vi "test Update Discrete Bit Field by Data Type.vi"(8 "error in (no error)":errorcluster, 11 "TestCase in":refnum<class "Discrete.lvclass">) -> (0 "error out":errorcluster, 3 "TestCase out":refnum<class "Discrete.lvclass">)   [LabVIEW 2027, in "Discrete.lvclass"]
uses:
  Discrete.lvclass
  6e1d2ac8-71cc-41db-b083-493d6063b283.vi
  b2aaa37d-0322-432e-9b3a-1a1fc6048de9.vi
  93c23f9b-5cd3-4544-9818-cc1d3354fe3b.vi
  d5bea4d0-148e-442b-ba51-e57cfb69b26e.vi
  0a8c8d56-0a15-4b3b-b00b-207fe3918b86.vi
  2c49008a-66d3-44d5-b62f-9e3dae6c920e.vi
  4d7c551b-64cf-497b-b044-69caef92442e.vi
  8e8a66e8-53e0-4356-8f39-caffdde6a543.vi
  751b3aa0-6cbc-42a9-8f45-cac4046d3a07.vi
  c0b90d40-c6d8-43ae-bb04-9b0646120204.vi
  7f187975-33e1-49fe-bcee-bbe8f41f89f8.vi
  20f2966f-f599-41d1-9ff8-715ba5da5165.vi
  6e1d2ac8-71cc-41db-b083-493d6063b283.vi/9935dc85-f143-411c-b80b-16b6c96eb14a.vi
  6e1d2ac8-71cc-41db-b083-493d6063b283.vi/b24d9be9-5807-4d59-88b8-dc532f996cb3.vi
  6e1d2ac8-71cc-41db-b083-493d6063b283.vi/e4a2156f-f189-4bbd-8a3a-9da1a7e591f8.vi
  b2aaa37d-0322-432e-9b3a-1a1fc6048de9.vi/9935dc85-f143-411c-b80b-16b6c96eb14a.vi
  b2aaa37d-0322-432e-9b3a-1a1fc6048de9.vi/b24d9be9-5807-4d59-88b8-dc532f996cb3.vi
  b2aaa37d-0322-432e-9b3a-1a1fc6048de9.vi/e4a2156f-f189-4bbd-8a3a-9da1a7e591f8.vi
  93c23f9b-5cd3-4544-9818-cc1d3354fe3b.vi/9935dc85-f143-411c-b80b-16b6c96eb14a.vi
  93c23f9b-5cd3-4544-9818-cc1d3354fe3b.vi/b24d9be9-5807-4d59-88b8-dc532f996cb3.vi
  93c23f9b-5cd3-4544-9818-cc1d3354fe3b.vi/e4a2156f-f189-4bbd-8a3a-9da1a7e591f8.vi
  d5bea4d0-148e-442b-ba51-e57cfb69b26e.vi/9935dc85-f143-411c-b80b-16b6c96eb14a.vi
  d5bea4d0-148e-442b-ba51-e57cfb69b26e.vi/b24d9be9-5807-4d59-88b8-dc532f996cb3.vi
  d5bea4d0-148e-442b-ba51-e57cfb69b26e.vi/e4a2156f-f189-4bbd-8a3a-9da1a7e591f8.vi
  0a8c8d56-0a15-4b3b-b00b-207fe3918b86.vi/9935dc85-f143-411c-b80b-16b6c96eb14a.vi
  0a8c8d56-0a15-4b3b-b00b-207fe3918b86.vi/b24d9be9-5807-4d59-88b8-dc532f996cb3.vi
  0a8c8d56-0a15-4b3b-b00b-207fe3918b86.vi/e4a2156f-f189-4bbd-8a3a-9da1a7e591f8.vi
  2c49008a-66d3-44d5-b62f-9e3dae6c920e.vi/9935dc85-f143-411c-b80b-16b6c96eb14a.vi
  2c49008a-66d3-44d5-b62f-9e3dae6c920e.vi/b24d9be9-5807-4d59-88b8-dc532f996cb3.vi
  2c49008a-66d3-44d5-b62f-9e3dae6c920e.vi/e4a2156f-f189-4bbd-8a3a-9da1a7e591f8.vi
  4d7c551b-64cf-497b-b044-69caef92442e.vi/9935dc85-f143-411c-b80b-16b6c96eb14a.vi
  4d7c551b-64cf-497b-b044-69caef92442e.vi/b24d9be9-5807-4d59-88b8-dc532f996cb3.vi
  4d7c551b-64cf-497b-b044-69caef92442e.vi/e4a2156f-f189-4bbd-8a3a-9da1a7e591f8.vi
  8e8a66e8-53e0-4356-8f39-caffdde6a543.vi/9935dc85-f143-411c-b80b-16b6c96eb14a.vi
  8e8a66e8-53e0-4356-8f39-caffdde6a543.vi/b24d9be9-5807-4d59-88b8-dc532f996cb3.vi
  8e8a66e8-53e0-4356-8f39-caffdde6a543.vi/e4a2156f-f189-4bbd-8a3a-9da1a7e591f8.vi
  751b3aa0-6cbc-42a9-8f45-cac4046d3a07.vi/9935dc85-f143-411c-b80b-16b6c96eb14a.vi
  751b3aa0-6cbc-42a9-8f45-cac4046d3a07.vi/b24d9be9-5807-4d59-88b8-dc532f996cb3.vi
  751b3aa0-6cbc-42a9-8f45-cac4046d3a07.vi/e4a2156f-f189-4bbd-8a3a-9da1a7e591f8.vi
  c0b90d40-c6d8-43ae-bb04-9b0646120204.vi/9935dc85-f143-411c-b80b-16b6c96eb14a.vi
  c0b90d40-c6d8-43ae-bb04-9b0646120204.vi/b24d9be9-5807-4d59-88b8-dc532f996cb3.vi
  c0b90d40-c6d8-43ae-bb04-9b0646120204.vi/e4a2156f-f189-4bbd-8a3a-9da1a7e591f8.vi
  7f187975-33e1-49fe-bcee-bbe8f41f89f8.vi/9935dc85-f143-411c-b80b-16b6c96eb14a.vi
  7f187975-33e1-49fe-bcee-bbe8f41f89f8.vi/b24d9be9-5807-4d59-88b8-dc532f996cb3.vi
  7f187975-33e1-49fe-bcee-bbe8f41f89f8.vi/e4a2156f-f189-4bbd-8a3a-9da1a7e591f8.vi
  20f2966f-f599-41d1-9ff8-715ba5da5165.vi/9935dc85-f143-411c-b80b-16b6c96eb14a.vi
  20f2966f-f599-41d1-9ff8-715ba5da5165.vi/b24d9be9-5807-4d59-88b8-dc532f996cb3.vi
  20f2966f-f599-41d1-9ff8-715ba5da5165.vi/e4a2156f-f189-4bbd-8a3a-9da1a7e591f8.vi
  C:/Program Files/National Instruments/LabVIEW 2027/vi.lib/addons/_JKI Toolkits/VI Tester/TestCase.llb/TestCase.lvclass
  <vilib>/addons/_JKI Toolkits/VI Tester/TestCase.llb/TestCase.lvclass
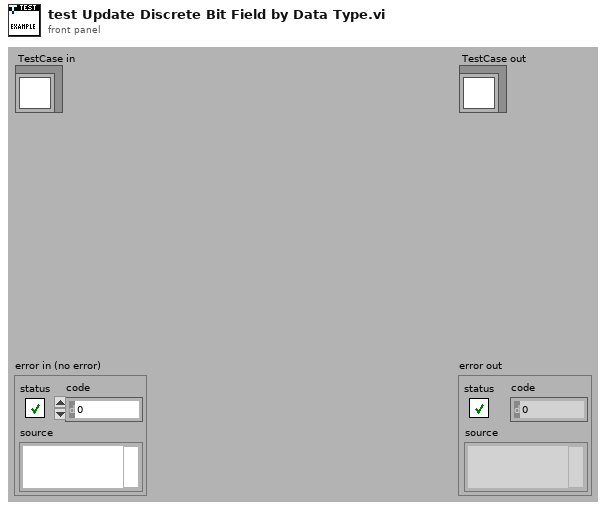
[diagram p1: front panel]
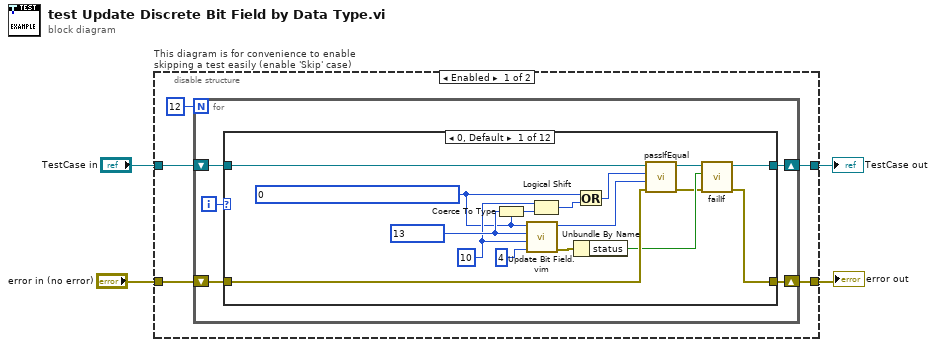
[diagram p0: block diagram]
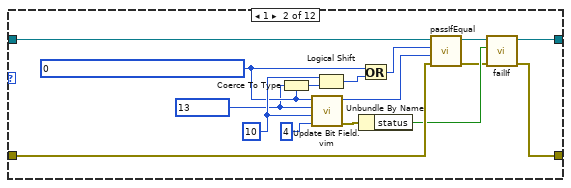
[diagram p2: hidden frame]
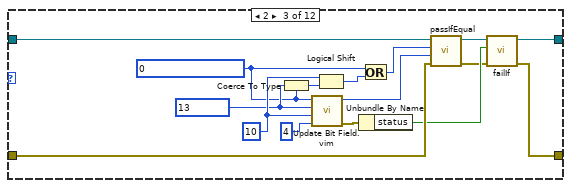
[diagram p3: hidden frame]
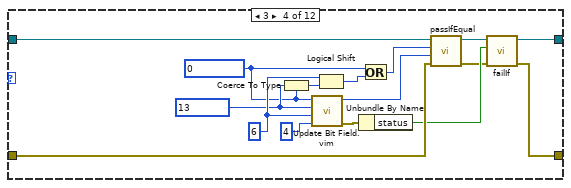
[diagram p4: hidden frame]
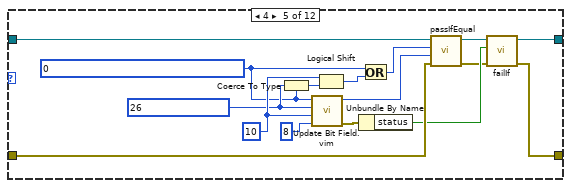
[diagram p5: hidden frame]
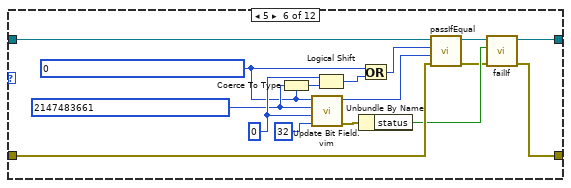
[diagram p6: hidden frame]
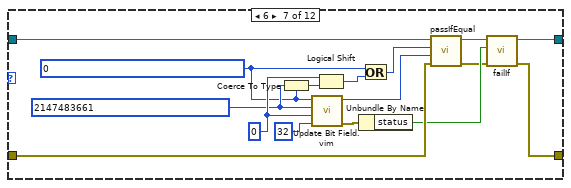
[diagram p7: hidden frame]
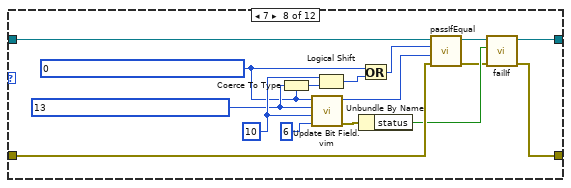
[diagram p8: hidden frame]
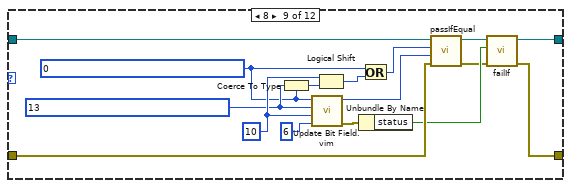
[diagram p9: hidden frame]
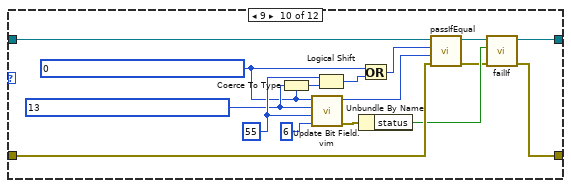
[diagram p10: hidden frame]
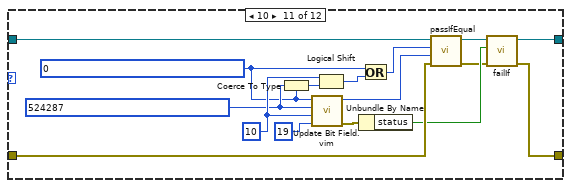
[diagram p11: hidden frame]
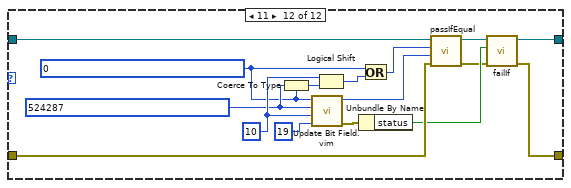
[diagram p12: hidden frame]
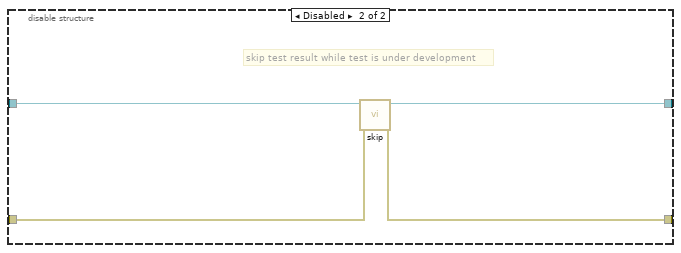
[diagram p13: hidden frame]
diagram:
  n1 = disable-structure "This diagram is for convenience to enable skipping a test easily (enable 'Skip' case)" shown="Enabled" {
    disable-tunnel: "TestCase in" -> [w9 w210]
    disable-tunnel: [w6 w208] -> w1
    disable-tunnel: [w7 w209] -> w3
    disable-tunnel: "error in (no error)" -> [w8 w207]
    frame Enabled {
      n2 = for {
        N: 12 -> [_]
        shift-right: [w11] -> w6
        shift-left: w9 -> [w14]
        shift-right: [w12] -> w7
        shift-left: w8 -> [w13]
        i -> [w10]
        n3 = case shown="0, Default" w10 {
          tunnel: w14 -> [w30 w46 w62 w78 w94 w110 w126 w142 w158 w174 w190 w206]
          tunnel: w13 -> [w29 w45 w61 w77 w93 w109 w125 w141 w157 w173 w189 w205]
          tunnel: [w28 w44 w60 w76 w92 w108 w124 w140 w156 w172 w188 w204] -> w12
          tunnel: [w27 w43 w59 w75 w91 w107 w123 w139 w155 w171 w187 w203] -> w11
          frame 0, Default {
            w18 = 10 ("bit field start index")
            w15 = u32 0 ("word in")
            w19 = u8 13 ("value")
            n4 = Coerce To Type(0:w19, 1:w15) -> (2:w17:u32)
            n5 = call "Update Bit Field.vim"("bit field size"=4, "bit field start index"=w18, "value"=w19, "word in"=w15) -> ("error out"=w23:errorcluster, "word out"=w24:u32)  [unwired: 6 in]
            n6 = Logical Shift(y=w18, x=w17) -> (x << y=w16:u32)
            n7 = Unbundle By Name(w23) -> ("status"=w22:bool)
            n8 = Or(x=w15, y=w16) -> (x .or. y?=w25:u32)
            n9 = call-dynamic "passIfEqual.vi"("error in (no error)"=w29, "y"=w24, "x"=w25, "TestCase in"=w30) -> ("error out"=w20:errorcluster, "TestCase out"=w21:refnum<class "Discrete.lvclass">)  [unwired: 6 in]
            n10 = call-dynamic "failIf.vi"("error in (no error)"=w20, "fail"=w22, "TestCase in"=w21) -> ("error out"=w28:errorcluster, "TestCase out"=w27:refnum<class "Discrete.lvclass">)  [unwired: 7 in]
          }
          frame 1 {
            w33 = 10 ("bit field start index")
            w32 = u64 0 ("word in")
            w31 = u8 13 ("value")
            n11 = Coerce To Type(0:w31, 1:w32) -> (2:w35:u64)
            n12 = call "Update Bit Field.vim"("bit field size"=4, "bit field start index"=w33, "value"=w31, "word in"=w32) -> ("error out"=w39:errorcluster, "word out"=w40:u64)  [unwired: 6 in]
            n13 = Logical Shift(y=w33, x=w35) -> (x << y=w34:u64)
            n14 = Unbundle By Name(w39) -> ("status"=w38:bool)
            n15 = Or(x=w32, y=w34) -> (x .or. y?=w41:u64)
            n16 = call-dynamic "passIfEqual.vi"("error in (no error)"=w45, "y"=w40, "x"=w41, "TestCase in"=w46) -> ("error out"=w36:errorcluster, "TestCase out"=w37:refnum<class "Discrete.lvclass">)  [unwired: 6 in]
            n17 = call-dynamic "failIf.vi"("error in (no error)"=w36, "fail"=w38, "TestCase in"=w37) -> ("error out"=w44:errorcluster, "TestCase out"=w43:refnum<class "Discrete.lvclass">)  [unwired: 7 in]
          }
          frame 2 {
            w49 = 10 ("bit field start index")
            w47 = u16 0 ("word in")
            w48 = u8 13 ("value")
            n18 = Coerce To Type(0:w48, 1:w47) -> (2:w51:u16)
            n19 = call "Update Bit Field.vim"("bit field size"=4, "bit field start index"=w49, "value"=w48, "word in"=w47) -> ("error out"=w55:errorcluster, "word out"=w56:u16)  [unwired: 6 in]
            n20 = Logical Shift(y=w49, x=w51) -> (x << y=w50:u16)
            n21 = Unbundle By Name(w55) -> ("status"=w54:bool)
            n22 = Or(x=w47, y=w50) -> (x .or. y?=w57:u16)
            n23 = call-dynamic "passIfEqual.vi"("error in (no error)"=w61, "y"=w56, "x"=w57, "TestCase in"=w62) -> ("error out"=w52:errorcluster, "TestCase out"=w53:refnum<class "Discrete.lvclass">)  [unwired: 6 in]
            n24 = call-dynamic "failIf.vi"("error in (no error)"=w52, "fail"=w54, "TestCase in"=w53) -> ("error out"=w60:errorcluster, "TestCase out"=w59:refnum<class "Discrete.lvclass">)  [unwired: 7 in]
          }
          frame 3 {
            w65 = 6 ("bit field start index")
            w63 = u8 0 ("word in")
            w64 = u8 13 ("value")
            n25 = Coerce To Type(0:w64, 1:w63) -> (2:w67:u8)
            n26 = call "Update Bit Field.vim"("bit field size"=4, "bit field start index"=w65, "value"=w64, "word in"=w63) -> ("error out"=w71:errorcluster, "word out"=w72:u8)  [unwired: 6 in]
            n27 = Logical Shift(y=w65, x=w67) -> (x << y=w66:u8)
            n28 = Unbundle By Name(w71) -> ("status"=w70:bool)
            n29 = Or(x=w63, y=w66) -> (x .or. y?=w73:u8)
            n30 = call-dynamic "passIfEqual.vi"("error in (no error)"=w77, "y"=w72, "x"=w73, "TestCase in"=w78) -> ("error out"=w68:errorcluster, "TestCase out"=w69:refnum<class "Discrete.lvclass">)  [unwired: 6 in]
            n31 = call-dynamic "failIf.vi"("error in (no error)"=w68, "fail"=w70, "TestCase in"=w69) -> ("error out"=w76:errorcluster, "TestCase out"=w75:refnum<class "Discrete.lvclass">)  [unwired: 7 in]
          }
          frame 4 {
            w81 = 10 ("bit field start index")
            w79 = u32 0 ("word in")
            w80 = u16 26 ("value")
            n32 = Coerce To Type(0:w80, 1:w79) -> (2:w83:u32)
            n33 = call "Update Bit Field.vim"("bit field size"=8, "bit field start index"=w81, "value"=w80, "word in"=w79) -> ("error out"=w87:errorcluster, "word out"=w88:u32)  [unwired: 6 in]
            n34 = Logical Shift(y=w81, x=w83) -> (x << y=w82:u32)
            n35 = Unbundle By Name(w87) -> ("status"=w86:bool)
            n36 = Or(x=w79, y=w82) -> (x .or. y?=w89:u32)
            n37 = call-dynamic "passIfEqual.vi"("error in (no error)"=w93, "y"=w88, "x"=w89, "TestCase in"=w94) -> ("error out"=w84:errorcluster, "TestCase out"=w85:refnum<class "Discrete.lvclass">)  [unwired: 6 in]
            n38 = call-dynamic "failIf.vi"("error in (no error)"=w84, "fail"=w86, "TestCase in"=w85) -> ("error out"=w92:errorcluster, "TestCase out"=w91:refnum<class "Discrete.lvclass">)  [unwired: 7 in]
          }
          frame 5 {
            w97 = 0 ("bit field start index")
            w95 = u32 0 ("word in")
            w96 = u32 2147483661 ("value")
            n39 = Coerce To Type(0:w96, 1:w95) -> (2:w99:u32)
            n40 = call "Update Bit Field.vim"("bit field size"=32, "bit field start index"=w97, "value"=w96, "word in"=w95) -> ("error out"=w103:errorcluster, "word out"=w104:u32)  [unwired: 6 in]
            n41 = Logical Shift(y=w97, x=w99) -> (x << y=w98:u32)
            n42 = Unbundle By Name(w103) -> ("status"=w102:bool)
            n43 = Or(x=w95, y=w98) -> (x .or. y?=w105:u32)
            n44 = call-dynamic "passIfEqual.vi"("error in (no error)"=w109, "y"=w104, "x"=w105, "TestCase in"=w110) -> ("error out"=w100:errorcluster, "TestCase out"=w101:refnum<class "Discrete.lvclass">)  [unwired: 6 in]
            n45 = call-dynamic "failIf.vi"("error in (no error)"=w100, "fail"=w102, "TestCase in"=w101) -> ("error out"=w108:errorcluster, "TestCase out"=w107:refnum<class "Discrete.lvclass">)  [unwired: 7 in]
          }
          frame 6 {
            w113 = 0 ("bit field start index")
            w111 = u32 0 ("word in")
            w112 = u64 2147483661 ("value")
            n46 = Coerce To Type(0:w112, 1:w111) -> (2:w115:u32)
            n47 = call "Update Bit Field.vim"("bit field size"=32, "bit field start index"=w113, "value"=w112, "word in"=w111) -> ("error out"=w119:errorcluster, "word out"=w120:u32)  [unwired: 6 in]
            n48 = Logical Shift(y=w113, x=w115) -> (x << y=w114:u32)
            n49 = Unbundle By Name(w119) -> ("status"=w118:bool)
            n50 = Or(x=w111, y=w114) -> (x .or. y?=w121:u32)
            n51 = call-dynamic "passIfEqual.vi"("error in (no error)"=w125, "y"=w120, "x"=w121, "TestCase in"=w126) -> ("error out"=w116:errorcluster, "TestCase out"=w117:refnum<class "Discrete.lvclass">)  [unwired: 6 in]
            n52 = call-dynamic "failIf.vi"("error in (no error)"=w116, "fail"=w118, "TestCase in"=w117) -> ("error out"=w124:errorcluster, "TestCase out"=w123:refnum<class "Discrete.lvclass">)  [unwired: 7 in]
          }
          frame 7 {
            w129 = 10 ("bit field start index")
            w127 = u32 0 ("word in")
            w128 = u64 13 ("value")
            n53 = Coerce To Type(0:w128, 1:w127) -> (2:w131:u32)
            n54 = call "Update Bit Field.vim"("bit field size"=6, "bit field start index"=w129, "value"=w128, "word in"=w127) -> ("error out"=w135:errorcluster, "word out"=w136:u32)  [unwired: 6 in]
            n55 = Logical Shift(y=w129, x=w131) -> (x << y=w130:u32)
            n56 = Unbundle By Name(w135) -> ("status"=w134:bool)
            n57 = Or(x=w127, y=w130) -> (x .or. y?=w137:u32)
            n58 = call-dynamic "passIfEqual.vi"("error in (no error)"=w141, "y"=w136, "x"=w137, "TestCase in"=w142) -> ("error out"=w132:errorcluster, "TestCase out"=w133:refnum<class "Discrete.lvclass">)  [unwired: 6 in]
            n59 = call-dynamic "failIf.vi"("error in (no error)"=w132, "fail"=w134, "TestCase in"=w133) -> ("error out"=w140:errorcluster, "TestCase out"=w139:refnum<class "Discrete.lvclass">)  [unwired: 7 in]
          }
          frame 8 {
            w145 = 10 ("bit field start index")
            w143 = u64 0 ("word in")
            w144 = u64 13 ("value")
            n60 = Coerce To Type(0:w144, 1:w143) -> (2:w147:u64)
            n61 = call "Update Bit Field.vim"("bit field size"=6, "bit field start index"=w145, "value"=w144, "word in"=w143) -> ("error out"=w151:errorcluster, "word out"=w152:u64)  [unwired: 6 in]
            n62 = Logical Shift(y=w145, x=w147) -> (x << y=w146:u64)
            n63 = Unbundle By Name(w151) -> ("status"=w150:bool)
            n64 = Or(x=w143, y=w146) -> (x .or. y?=w153:u64)
            n65 = call-dynamic "passIfEqual.vi"("error in (no error)"=w157, "y"=w152, "x"=w153, "TestCase in"=w158) -> ("error out"=w148:errorcluster, "TestCase out"=w149:refnum<class "Discrete.lvclass">)  [unwired: 6 in]
            n66 = call-dynamic "failIf.vi"("error in (no error)"=w148, "fail"=w150, "TestCase in"=w149) -> ("error out"=w156:errorcluster, "TestCase out"=w155:refnum<class "Discrete.lvclass">)  [unwired: 7 in]
          }
          frame 9 {
            w161 = 55 ("bit field start index")
            w159 = u64 0 ("word in")
            w160 = u64 13 ("value")
            n67 = Coerce To Type(0:w160, 1:w159) -> (2:w163:u64)
            n68 = call "Update Bit Field.vim"("bit field size"=6, "bit field start index"=w161, "value"=w160, "word in"=w159) -> ("error out"=w167:errorcluster, "word out"=w168:u64)  [unwired: 6 in]
            n69 = Logical Shift(y=w161, x=w163) -> (x << y=w162:u64)
            n70 = Unbundle By Name(w167) -> ("status"=w166:bool)
            n71 = Or(x=w159, y=w162) -> (x .or. y?=w169:u64)
            n72 = call-dynamic "passIfEqual.vi"("error in (no error)"=w173, "y"=w168, "x"=w169, "TestCase in"=w174) -> ("error out"=w164:errorcluster, "TestCase out"=w165:refnum<class "Discrete.lvclass">)  [unwired: 6 in]
            n73 = call-dynamic "failIf.vi"("error in (no error)"=w164, "fail"=w166, "TestCase in"=w165) -> ("error out"=w172:errorcluster, "TestCase out"=w171:refnum<class "Discrete.lvclass">)  [unwired: 7 in]
          }
          frame 10 {
            w177 = 10 ("bit field start index")
            w175 = u32 0 ("word in")
            w176 = u64 524287 ("value")
            n74 = Coerce To Type(0:w176, 1:w175) -> (2:w179:u32)
            n75 = call "Update Bit Field.vim"("bit field size"=19, "bit field start index"=w177, "value"=w176, "word in"=w175) -> ("error out"=w183:errorcluster, "word out"=w184:u32)  [unwired: 6 in]
            n76 = Logical Shift(y=w177, x=w179) -> (x << y=w178:u32)
            n77 = Unbundle By Name(w183) -> ("status"=w182:bool)
            n78 = Or(x=w175, y=w178) -> (x .or. y?=w185:u32)
            n79 = call-dynamic "passIfEqual.vi"("error in (no error)"=w189, "y"=w184, "x"=w185, "TestCase in"=w190) -> ("error out"=w180:errorcluster, "TestCase out"=w181:refnum<class "Discrete.lvclass">)  [unwired: 6 in]
            n80 = call-dynamic "failIf.vi"("error in (no error)"=w180, "fail"=w182, "TestCase in"=w181) -> ("error out"=w188:errorcluster, "TestCase out"=w187:refnum<class "Discrete.lvclass">)  [unwired: 7 in]
          }
          frame 11 {
            w193 = 10 ("bit field start index")
            w191 = u32 0 ("word in")
            w192 = u32 524287 ("value")
            n81 = Coerce To Type(0:w192, 1:w191) -> (2:w195:u32)
            n82 = call "Update Bit Field.vim"("bit field size"=19, "bit field start index"=w193, "value"=w192, "word in"=w191) -> ("error out"=w199:errorcluster, "word out"=w200:u32)  [unwired: 6 in]
            n83 = Logical Shift(y=w193, x=w195) -> (x << y=w194:u32)
            n84 = Unbundle By Name(w199) -> ("status"=w198:bool)
            n85 = Or(x=w191, y=w194) -> (x .or. y?=w201:u32)
            n86 = call-dynamic "passIfEqual.vi"("error in (no error)"=w205, "y"=w200, "x"=w201, "TestCase in"=w206) -> ("error out"=w196:errorcluster, "TestCase out"=w197:refnum<class "Discrete.lvclass">)  [unwired: 6 in]
            n87 = call-dynamic "failIf.vi"("error in (no error)"=w196, "fail"=w198, "TestCase in"=w197) -> ("error out"=w204:errorcluster, "TestCase out"=w203:refnum<class "Discrete.lvclass">)  [unwired: 7 in]
          }
        }
      }
    }
    frame Disabled {
      # "skip test result while test is under development"
      n88 = call <vilib>:"skip.vi"("error in (no error)"=w207, "TestCase in"=w210) -> ("error out"=w209:errorcluster, "TestCase out"=w208:refnum<class "Discrete.lvclass">)  [unwired: 8 in]
    }
  }
  "error out" <- w3
  "TestCase out" <- w1
